vi "Write Score Data To File.vi"(10 "XML File Path":path) -> (2 "XML":string)   [LabVIEW 2013]
uses:
  <vilib>/xml/Close Reference(Node).vi
  <vilib>/xml/NI_XML.lvlib
  <resource>/objmgr/DOMUserDefRef.rc
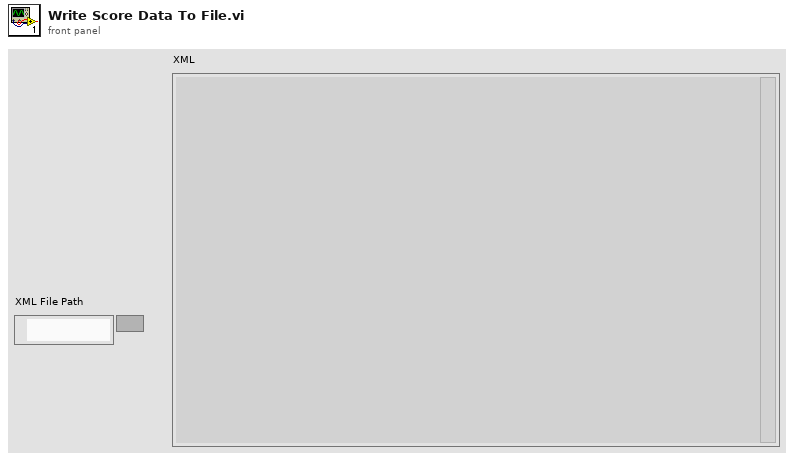
[diagram p1: front panel]
types:
  T1 = typedef "ScoreList.ctl" = cluster{"ValidationCount":u16, "Score":T2}[]
  T2 = typedef "Full Score Entry.ctl" = cluster{"GUID":u16, "Score Mode Selector":u16, "Round Number":u16, "Full Score Entry":T3}
  T3 = typedef "ScoreEntry.ctl" = cluster{"Elements":cluster{"Name":string, "Value":string}[], "Score":dbl}
  T4 = cluster{"Both":string, "Name":string, "GUID":u16, "Number":u16}
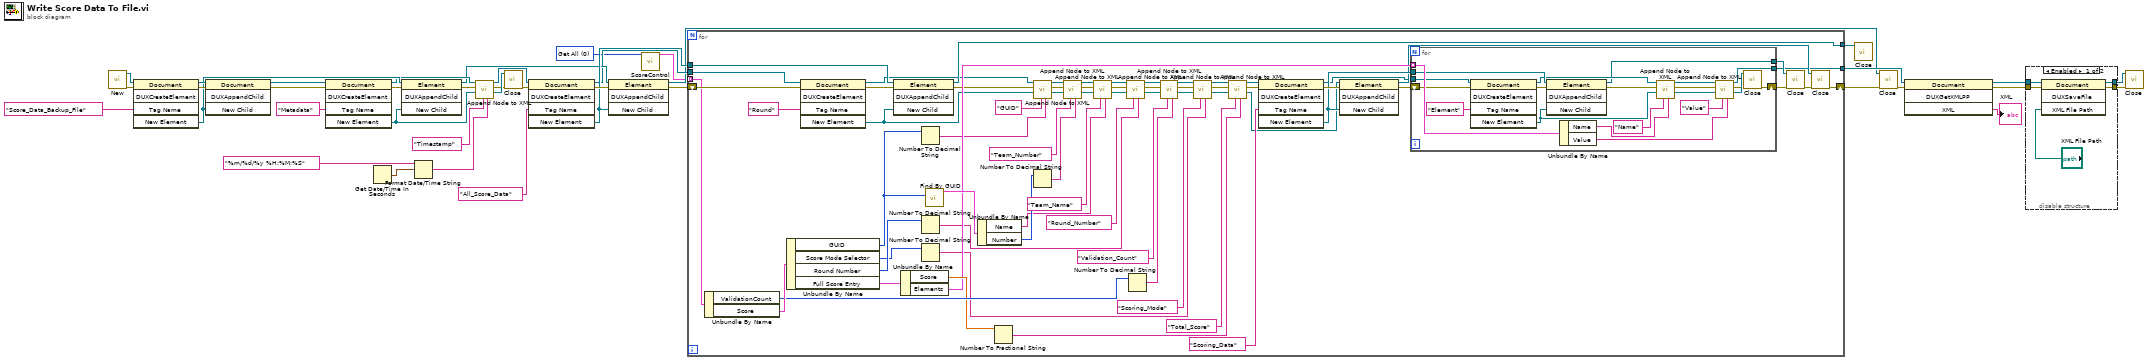
[diagram p0: block diagram]
diagram:
  w2 = u16 0 items=["Get All", "Set", "Reset All", "Force Set"] ("Get/Set Mode Selector")
  n1 = call <vilib>:"New.vi"() -> ("error out"=w24:errorcluster, "DOM document out"=w25:refnum<k20>)  [unwired: 8 in]
  n2 = invoke class="Document" method="DUXCreateElement"(reference=w25, error in=w24, "Tag Name"="Score_Data_Backup_File") -> (reference out=w22:refnum<k20>, error out=w21:errorcluster, "New Element"=w18:refnum<k20>)  [unwired: 2 in, 2 out]
  n3 = invoke class="Document" method="DUXAppendChild"(reference=w22, error in=w21, "New Child"=w18) -> (reference out=w20:refnum<k20>, error out=w19:errorcluster)  [unwired: 1 in, 2 out]
  n4 = invoke class="Document" method="DUXCreateElement"(reference=w20, error in=w19, "Tag Name"="Metadata") -> (reference out=w17:refnum<k20>, error out=w36:errorcluster, "New Element"=w3:refnum<k20>)  [unwired: 2 in, 2 out]
  n5 = Get Date/Time In Seconds() -> (seconds since 1Jan1904=w33:timestamp)
  n6 = invoke class="Element" method="DUXAppendChild"(reference=w18, error in=w36, "New Child"=w3) -> (reference out=w16:refnum<k20>, error out=w35:errorcluster)  [unwired: 1 in, 2 out]
  n7 = Format Date/Time String(time format string (%c)="%m/%d/%y %H:%M:%S", seconds (now)=w33) -> (date/time string=w5:string)  [unwired: 1 in]
  n8 = call "Append Node to XML.vi"("Data"=w5, "Tag Name"="Timestamp", "SuperElement In"=w3, "error in"=w35, "DOM document in"=w17) -> ("SuperElement Out"=w31:refnum<k20>, "error out"=w30:errorcluster, "DOM document out"=w34:refnum<k20>)  [unwired: 4 in]
  n9 = call-poly <vilib>:"Close.vi"("error in (no error)"=w30, "node"=w31) -> ("error out"=w14:errorcluster)  [unwired: 7 in]
  n10 = invoke class="Document" method="DUXCreateElement"(reference=w34, error in=w14, "Tag Name"="All_Score_Data") -> (reference out=w15:refnum<k20>, error out=w39:errorcluster, "New Element"=w29:refnum<k20>)  [unwired: 2 in, 2 out]
  n11 = invoke class="Element" method="DUXAppendChild"(reference=w16, error in=w39, "New Child"=w29) -> (reference out=w12:refnum<k20>, error out=w13:errorcluster)  [unwired: 1 in, 2 out]
  n12 = call "ScoreControl.vi"("Get/Set Mode Selector"=w2) -> ("Scores"=w1:T1)  [unwired: 13 in, 1 out]
  n13 = for {
    tunnel: w1 -> [w102] mode=indexing
    tunnel: w15 -> [w105]
    shift-right: [w71] -> w11
    shift-left: w13 -> [w104]
    tunnel: w29 -> [w73]
    tunnel: [w72] -> w28
    tunnel: [w70] -> w26
    n14 = Unbundle By Name(w102) -> ("ValidationCount"=w89:u16, "Score"=w101:T2)
    n15 = Unbundle By Name(w101) -> ("GUID"=w100:u16, "Score Mode Selector"=w86:u16, "Round Number"=w92:u16, "Full Score Entry"=w83:T3)
    n16 = invoke class="Document" method="DUXCreateElement"(reference=w105, error in=w104, "Tag Name"="Round") -> (reference out=w47:refnum<k20>, error out=w69:errorcluster, "New Element"=w44:refnum<k20>)  [unwired: 2 in, 2 out]
    n17 = invoke class="Element" method="DUXAppendChild"(reference=w73, error in=w69, "New Child"=w44) -> (reference out=w72:refnum<k20>, error out=w45:errorcluster)  [unwired: 1 in, 2 out]
    n18 = Unbundle By Name(w83) -> ("Score"=w82:dbl, "Elements"=w79:cluster{"Name":string, "Value":string}[])
    n19 = Number To Decimal String(number=w100) -> (decimal integer string=w67:string)  [unwired: 1 in]
    n20 = Number To Decimal String(number=w92) -> (decimal integer string=w57:string)  [unwired: 1 in]
    n21 = Number To Decimal String(number=w86) -> (decimal integer string=w51:string)  [unwired: 1 in]
    n22 = call "Find By GUID.vi"("GUID"=w100) -> ("Team"=w97:T4)  [unwired: 9 in, 1 out]
    n23 = Unbundle By Name(w97) -> ("Name"=w61:string, "Number"=w96:u16)
    n24 = Number To Fractional String(number=w82) -> (F-format string=w48:string)  [unwired: 3 in]
    n25 = call "Append Node to XML.vi"("Data"=w67, "Tag Name"="GUID", "SuperElement In"=w44, "error in"=w45, "DOM document in"=w47) -> ("SuperElement Out"=w66:refnum<k20>, "error out"=w98:errorcluster, "DOM document out"=w99:refnum<k20>)  [unwired: 4 in]
    n26 = Number To Decimal String(number=w96) -> (decimal integer string=w64:string)  [unwired: 1 in]
    n27 = call "Append Node to XML.vi"("Data"=w64, "Tag Name"="Team_Number", "SuperElement In"=w66, "error in"=w98, "DOM document in"=w99) -> ("SuperElement Out"=w63:refnum<k20>, "error out"=w95:errorcluster, "DOM document out"=w94:refnum<k20>)  [unwired: 4 in]
    n28 = call "Append Node to XML.vi"("Data"=w61, "Tag Name"="Team_Name", "SuperElement In"=w63, "error in"=w95, "DOM document in"=w94) -> ("SuperElement Out"=w60:refnum<k20>, "error out"=w59:errorcluster, "DOM document out"=w93:refnum<k20>)  [unwired: 4 in]
    n29 = call "Append Node to XML.vi"("Data"=w57, "Tag Name"="Round_Number", "SuperElement In"=w60, "error in"=w59, "DOM document in"=w93) -> ("SuperElement Out"=w54:refnum<k20>, "error out"=w91:errorcluster, "DOM document out"=w90:refnum<k20>)  [unwired: 4 in]
    n30 = Number To Decimal String(number=w89) -> (decimal integer string=w55:string)  [unwired: 1 in]
    n31 = call "Append Node to XML.vi"("Data"=w55, "Tag Name"="Validation_Count", "SuperElement In"=w54, "error in"=w91, "DOM document in"=w90) -> ("SuperElement Out"=w53:refnum<k20>, "error out"=w87:errorcluster, "DOM document out"=w88:refnum<k20>)  [unwired: 4 in]
    n32 = call "Append Node to XML.vi"("Data"=w51, "Tag Name"="Scoring_Mode", "SuperElement In"=w53, "error in"=w87, "DOM document in"=w88) -> ("SuperElement Out"=w50:refnum<k20>, "error out"=w80:errorcluster, "DOM document out"=w81:refnum<k20>)  [unwired: 4 in]
    n33 = call "Append Node to XML.vi"("Data"=w48, "Tag Name"="Total_Score", "SuperElement In"=w50, "error in"=w80, "DOM document in"=w81) -> ("SuperElement Out"=w41:refnum<k20>, "error out"=w40:errorcluster, "DOM document out"=w42:refnum<k20>)  [unwired: 4 in]
    n34 = invoke class="Document" method="DUXCreateElement"(reference=w42, error in=w40, "Tag Name"="Scoring_Data") -> (reference out=w46:refnum<k20>, error out=w84:errorcluster, "New Element"=w78:refnum<k20>)  [unwired: 2 in, 2 out]
    n35 = invoke class="Element" method="DUXAppendChild"(reference=w41, error in=w84, "New Child"=w78) -> (reference out=w74:refnum<k20>, error out=w77:errorcluster)  [unwired: 1 in, 2 out]
    n36 = for {
      tunnel: w79 -> [w126] mode=indexing
      tunnel: w46 -> [w125]
      tunnel: w78 -> [w122]
      shift-right: [w114] -> w43
      shift-left: w77 -> [w124]
      tunnel: [w113] -> w76
      tunnel: [w112] -> w70
      n37 = invoke class="Document" method="DUXCreateElement"(reference=w125, error in=w124, "Tag Name"="Element") -> (reference out=w120:refnum<k20>, error out=w121:errorcluster, "New Element"=w106:refnum<k20>)  [unwired: 2 in, 2 out]
      n38 = invoke class="Element" method="DUXAppendChild"(reference=w122, error in=w121, "New Child"=w106) -> (reference out=w113:refnum<k20>, error out=w119:errorcluster)  [unwired: 1 in, 2 out]
      n39 = Unbundle By Name(w126) -> ("Name"=w107:string, "Value"=w109:string)
      n40 = call "Append Node to XML.vi"("Data"=w107, "Tag Name"="Name", "SuperElement In"=w106, "error in"=w119, "DOM document in"=w120) -> ("SuperElement Out"=w111:refnum<k20>, "error out"=w117:errorcluster, "DOM document out"=w118:refnum<k20>)  [unwired: 4 in]
      n41 = call "Append Node to XML.vi"("Data"=w109, "Tag Name"="Value", "SuperElement In"=w111, "error in"=w117, "DOM document in"=w118) -> ("SuperElement Out"=w116:refnum<k20>, "error out"=w115:errorcluster, "DOM document out"=w112:refnum<k20>)  [unwired: 4 in]
      n42 = call-poly <vilib>:"Close.vi"("error in (no error)"=w115, "node"=w116) -> ("error out"=w114:errorcluster)  [unwired: 7 in]
    }
    n43 = call-poly <vilib>:"Close.vi"("error in (no error)"=w43, "node"=w76) -> ("error out"=w75:errorcluster)  [unwired: 7 in]
    n44 = call-poly <vilib>:"Close.vi"("error in (no error)"=w75, "node"=w74) -> ("error out"=w71:errorcluster)  [unwired: 7 in]
  }
  n45 = call-poly <vilib>:"Close.vi"("node"=w28) -> ()  [unwired: 8 in, 1 out]
  n46 = call-poly <vilib>:"Close.vi"("error in (no error)"=w11, "node"=w12) -> ("error out"=w10:errorcluster)  [unwired: 7 in]
  n47 = invoke class="Document" method="DUXGetXMLPP"(reference=w26, error in=w10) -> (reference out=w9:refnum<k20>, error out=w8:errorcluster, "XML"=→"XML":string)  [unwired: 2 in, 1 out]
  n48 = disable-structure shown="Enabled" {
    disable-tunnel: w9 -> [w131 w133]
    disable-tunnel: w8 -> [w130 w132]
    disable-tunnel: [w128 w133] -> w7
    disable-tunnel: [w127 w132] -> w6
    frame Enabled {
      n49 = invoke class="Document" method="DUXSaveFile"(reference=w131, error in=w130, "XML File Path"="XML File Path") -> (reference out=w128:refnum<k20>, error out=w127:errorcluster)  [unwired: 1 in, 2 out]
    }
    frame Disabled {
    }
  }
  n50 = call-poly <vilib>:"Close.vi"("error in (no error)"=w6, "node"=w7) -> ()  [unwired: 7 in, 1 out]
